vi "1D array remove duplicates.vi"(11 "input array":dbl[](array[numeric])=[0.0, 0.0, 1.0, 3.0, 2.0, 3.0, 2.0, 1.0, 0.0]) -> (3 "output array":dbl[](array[numeric])=[0.0, 1.0, 3.0, 2.0])   [LabVIEW 2020]
panel:
  # "remove duplicate elements from 1D array"
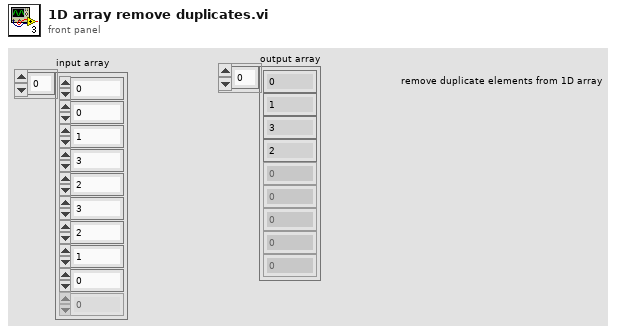
[diagram p1: front panel]
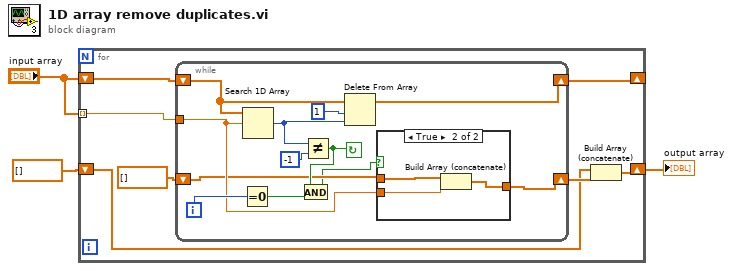
[diagram p0: block diagram]
diagram:
  n1 = for {
    tunnel: "input array" -> [w9] mode=indexing
    shift-right: [w7] -> _
    shift-left: "input array" -> [w10]
    shift-right: [w6] -> w1
    shift-left: dbl[] [] -> [w4]
    n2 = while {
      tunnel: w9 -> [w16]
      shift-right: [w15] -> w5
      shift-left: dbl[] [] -> [w14]
      shift-right: [w22] -> w7
      shift-left: w10 -> [w21]
      i -> [w19]
      stop <- w17 continue-if-true
      n3 = Equal To 0?(x=w19) -> (x = 0?=w18:bool)
      n4 = Search 1D Array(1D array=w21, element=w16) -> (index of element=w13:i32)  [unwired: 1 in]
      n5 = Not Equal?(x=w13, y=-1) -> (x != y?=w17:bool)
      n6 = And(x=w17, y=w18) -> (x .and. y?=w11:bool)
      n7 = Delete From Array(array=w21, length=1, index=w13) -> (array with subset deleted=w22:dbl[])  [unwired: 1 out]
      n8 = case shown="True" w11 {
        tunnel: w16 -> [_ w25]
        tunnel: [w23 w26] -> w15
        tunnel: w14 -> [w23 w24]
        frame False {
        }
        frame True {
          n9 = Build Array (concatenate)(w24, w25) -> (w26:dbl[])
        }
      }
    }
    n10 = Build Array (concatenate)(w4, w5) -> (w6:dbl[])
  }
  "output array" <- w1
